vi "Array1DLastNElements.vi"(2 "Array in":dbl[](array[numeric]), 3 "N":i32=950) -> (1 "Array out":dbl[](array[numeric]))   [LabVIEW 2014]
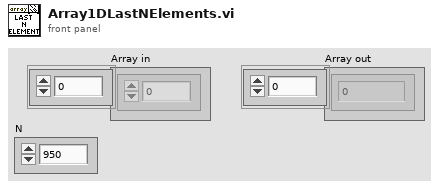
[diagram p1: front panel]
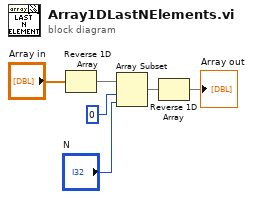
[diagram p0: block diagram]
diagram:
  n1 = Reverse 1D Array(array="Array in") -> (reversed array=w2:dbl[])
  n2 = Array Subset(array=w2, index=0, length="N") -> (w1:dbl[])
  n3 = Reverse 1D Array(array=w1) -> (reversed array=→"Array out":dbl[])
